vi "samp_s2_2019.vi"() -> ()   [LabVIEW 2021]
uses:
  Open_device_2018.llb/Select_Instr.ctl
panel:
  out "Voltage":dbl
  out "Read counter":i32
  out "error out":errorcluster
  out "Opened":bool
  in  "stop":bool
  out "read buffer":string
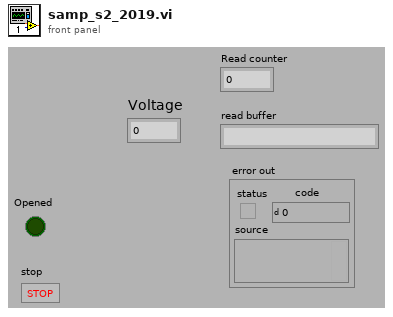
[diagram p1: front panel]
types:
  T1 = typedef "Select_Instr.ctl" = string
  T2 = cluster{"VISA resource name 1":refnum<visa-resource-name>, "VISA resource name 2":refnum<visa-resource-name>, "VISA resource name 3":refnum<visa-resource-name>}
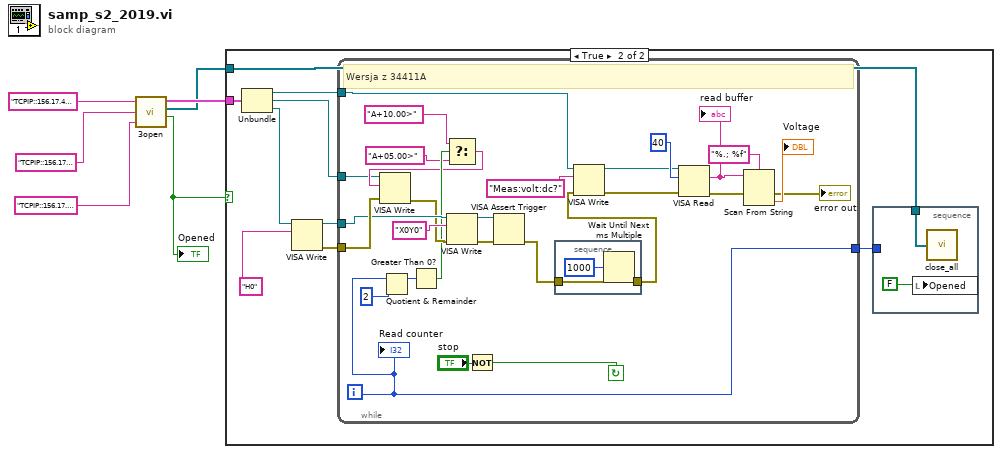
[diagram p0: block diagram]
diagram:
  n1 = call "3open.vi"("VISA resource name 1"=T1 "TCPIP::156.17.45.35::inst21::INSTR" ("Select_Instrument"), "VISA resource name 2"=T1 "TCPIP::156.17.45.35::inst18::INSTR" ("Select_Instrument"), "VISA resource name 3"=T1 "TCPIP::156.17.45.35::inst19::INSTR" ("Select_Instrument")) -> ("InstrCluster"=w6:T2, "InstrArray"=w5:refnum<visa-resource-name>[], "Open OK (true)"=w4:bool)  [unwired: 1 in, 1 out]
  "Opened" <- w4
  n2 = case shown="True" w4 {
    tunnel: w6 -> [_ w10]
    tunnel: w5 -> [_ w11]
    frame False {
    }
    frame True {
      n3 = Unbundle(w10) -> ("VISA resource name 1"=w7:refnum<visa-resource-name>, "VISA resource name 2"=w9:refnum<visa-resource-name>, "VISA resource name 3"=w8:refnum<visa-resource-name>)
      n4 = VISA Write(VISA resource name=w8, write buffer="H0" ("write buffer (\"\")")) -> (VISA resource name out=w14:refnum<visa-resource-name>, error out=w13:errorcluster)  [unwired: 1 in, 1 out]
      n5 = while {
        tunnel: [w32] -> w15
        tunnel: w14 -> [w37]
        tunnel: w13 -> [w38]
        tunnel: w9 -> [w26]
        tunnel: w7 -> [w20]
        i -> [w32]
        stop <- w42 continue-if-true
        # "Wersja z 34411A"
        n6 = Quotient & Remainder(x=w32, y=2) -> (x-y*floor(x/y)=w31:i32)  [unwired: 1 out]
        n7 = Greater Than 0?(x=w31) -> (x > 0?=w30:bool)
        n8 = Select(t="A+10.00>" ("write buffer (\"\")"), s=w30, f="A+05.00>") -> (s? t:f=w27:string)
        n9 = VISA Write(VISA resource name=w26, write buffer=w27, error in (no error)=w38) -> (error out=w36:errorcluster)  [unwired: 2 out]
        n10 = VISA Write(VISA resource name=w37, write buffer="X0Y0" ("write buffer (\"\")"), error in (no error)=w36) -> (VISA resource name out=w39:refnum<visa-resource-name>, error out=w40:errorcluster)  [unwired: 1 out]
        n11 = Not(x="stop") -> (.not. x?=w42:bool)
        n12 = VISA Assert Trigger(8:w40, 11:w39) -> (0:w35:errorcluster)  [unwired: 1 in, 1 out]
        n13 = stacked-sequence {
          tunnel: w35 -> [w46]
          tunnel: [w46] -> w34
          frame #0 {
            n14 = Wait Until Next ms Multiple(millisecond multiple=u32 1000) -> ()  [unwired: 1 out]
          }
        }
        n15 = VISA Write(VISA resource name=w20, write buffer="Meas:volt:dc?" ("write buffer (\"\")"), error in (no error)=w34) -> (VISA resource name out=w19:refnum<visa-resource-name>, error out=w18:errorcluster)  [unwired: 1 out]
        n16 = VISA Read(VISA resource name=w19, byte count=u32 40 ("byte count (0)"), error in (no error)=w18) -> (read buffer=w24:string, error out=w25:errorcluster)  [unwired: 2 out]
        "read buffer" <- w24
        n17 = Scan From String(format string="%.; %f", input string=w24, error in=w25) -> (error out=→"error out":errorcluster, output 1=→"Voltage":dbl)  [unwired: 2 in, 2 out]
        "Read counter" <- w32
      }
      n18 = stacked-sequence {
        tunnel: w15 -> [_]
        tunnel: w11 -> [w16]
        frame #0 {
          n19 = local write "Opened"(FALSE) -> ()
          n20 = call "close_all.vi"("OpenRes"=w16) -> ()  [unwired: 1 out]
        }
      }
    }
  }
